vi "方程子VI.vi"() -> ()   [LabVIEW 2018]
panel:
  out "输出变量":dbl
  in  "A":dbl
  in  "C":dbl
  in  "B":dbl
  in  "X":dbl
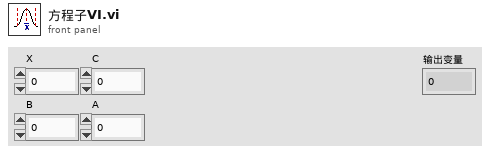
[diagram p1: front panel]
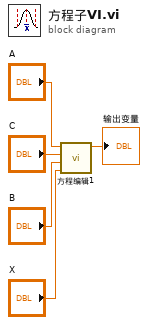
[diagram p0: block diagram]
diagram:
  n1 = call "方程编辑1.vi"("X"="X", "B"="B", "C"="C", "A"="A") -> ("输出变量"=→"输出变量":dbl)  [unwired: 7 in]
